vi "添加长度头.vi"(11 "cmd":string) -> (3 "添加后":string)   [LabVIEW 2015]
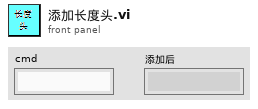
[diagram p1: front panel]
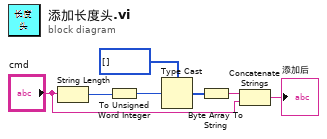
[diagram p0: block diagram]
diagram:
  n1 = String Length(string="cmd") -> (length=w3:i32)
  n2 = To Unsigned Word Integer(number=w3) -> (unsigned 16bit integer=w1:u16)
  n3 = Type Cast(type=u8[] [], x=w1) -> (*(type *) &x=w7:u8[])
  n4 = Byte Array To String(unsigned byte array=w7) -> (string=w4:string)
  n5 = Concatenate Strings(w4, "cmd") -> (→"添加后":string)
